vi "read_diode.vi"(9 "DAQmx Physical Channel":tag="cDAQ1Mod1/ai0") -> (1 "% Coupled":dbl)   [LabVIEW 2020]
uses:
  <vilib>/DAQmx/read.llb/DAQmx Read (Analog 1D Wfm NChan NSamp).vi
  <vilib>/Analysis/NI_AALBase.lvlib
  <vilib>/Analysis/baseanly.llb/Mean (DBL).vi
  <vilib>/DAQmx/create/channels.llb/DAQmx Create Channel (AI-Voltage-Basic).vi
  <vilib>/DAQmx/configure/timing.llb/DAQmx Timing (Sample Clock).vi
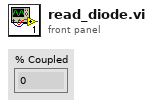
[diagram p1: front panel]
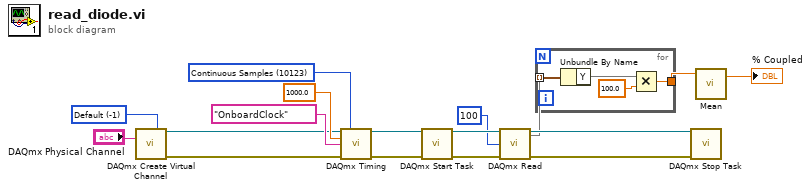
[diagram p0: block diagram]
diagram:
  w16 = -1 items=["Default"=-1, "RSE"=10083, "NRSE"=10078, "Differential"=10106, "Pseudodifferential"=12529] ("input terminal configuration")
  w17 = 10123 items=["Finite Samples"=10178, "Continuous Samples"=10123, "Hardware Timed Single Point"=12522] ("sample mode")
  n1 = call-poly <vilib>:"DAQmx Create Virtual Channel.vi"("input terminal configuration"=w16, "physical channels"="DAQmx Physical Channel") -> ("task out"=w12:refnum<k21>, "error out"=w13:errorcluster)  [unwired: 12 in]
  n2 = call-poly <vilib>:"DAQmx Timing.vi"("task/channels in"=w12, "sample mode"=w17, "rate"=1000.0 ("sample rate"), "source"=tag "OnboardClock", "error in"=w13) -> ("task out"=w10:refnum<k21>, "error out"=w9:errorcluster)  [unwired: 9 in]
  n3 = call <vilib>:"DAQmx Start Task.vi"("task/channels in"=w10, "error in"=w9) -> ("task out"=w5:refnum<k21>, "error out"=w6:errorcluster)  [unwired: 12 in]
  n4 = call-poly <vilib>:"DAQmx Read.vi"("task/channels in"=w5, "number of samples per channel"=100 ("n samples/channel"), "error in"=w6) -> (3:w3, "task out"=w7:refnum<k21>, "error out"=w8:errorcluster)  [unwired: 9 in, 1 out]
  n5 = for {
    tunnel: [w20] -> w2
    tunnel: w3 -> [w18] mode=indexing
    n6 = Unbundle By Name(w18) -> ("Y"=w19)
    n7 = Multiply(x=w19, y=100.0) -> (x*y=w20:dbl)
  }
  n8 = call <vilib>:"DAQmx Stop Task.vi"("task/channels in"=w7, "error in"=w8) -> ()  [unwired: 12 in, 2 out]
  n9 = call-poly <vilib>:"Mean.vi"("X"=w2) -> ("mean"=→"% Coupled":dbl)  [unwired: 1 out]
